vi "m1m3_putSample_HardpointMonitorData.vi"(8 "error in (no error)":errorcluster, 11 "HardpointMonitorData_Ctl":T1={"Timestamp"=0.0, "BreakawayLVDT[6]"=[0.0, 0.0, 0.0, 0.0, 0.0, 0.0], "DisplacementLVDT[6]"=[0.0, 0.0, 0.0, 0.0, 0.0, 0.0], "BreakawayPressure[6]"=[0.0, 0.0, 0.0, 0.0, 0.0, 0.0], "PressureSensor1[6]"=[0.0, 0.0, 0.0, 0.0, 0.0, 0.0], "PressureSensor2[6]"=[0.0, 0.0, 0.0, 0.0, 0.0, 0.0], "PressureSensor3[6]"=[0.0, 0.0, 0.0, 0.0, 0.0, 0.0]}) -> (0 "error out":errorcluster, 2 "function return":i32, 3 "HardpointMonitorData_Ctl out":T1)   [LabVIEW 2016, in "SALLV_m1m3.lvlib"]
doc: "int m1m3_shm_putSample_HardpointMonitorDataLV(m1m3_HardpointMonitorDataLV *HardpointMonitorData_Ctl );"
uses:
  SALLV_m1m3.lvlib
  DataTypes/HardpointMonitorData.ctl
  SALLV_m1m3.so
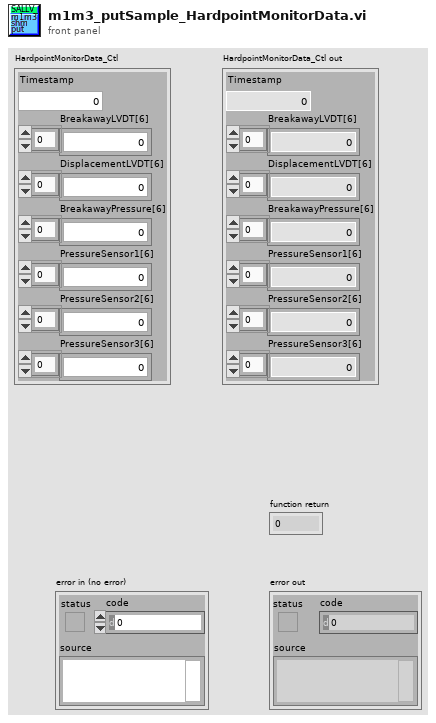
[diagram p1: front panel]
types:
  T1 = typedef "SALLV_m1m3.lvlib/HardpointMonitorData.ctl" = cluster{"Timestamp":dbl, "BreakawayLVDT[6]":sgl[], "DisplacementLVDT[6]":sgl[], "BreakawayPressure[6]":sgl[], "PressureSensor1[6]":sgl[], "PressureSensor2[6]":sgl[], "PressureSensor3[6]":sgl[]}
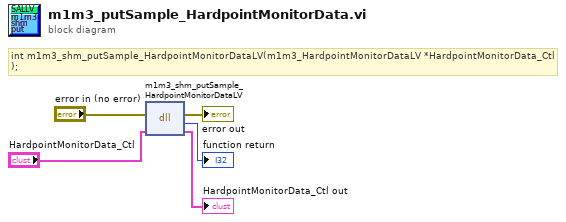
[diagram p0: block diagram]
diagram:
  # "int m1m3_shm_putSample_HardpointMonitorDataLV(m1m3_HardpointMonitorDataLV *HardpointMonitorData_Ctl );"
  n1 = dll-call lib="opt/CODE/SALLV_m1m3/SALLV_m1m3.*" fn="m1m3_shm_putSample_HardpointMonitorDataLV"(error in="error in (no error)", "HardpointMonitorData_Ctl"="HardpointMonitorData_Ctl") -> (error out=→"error out":errorcluster, →"function return":i32, "HardpointMonitorData_Ctl"=→"HardpointMonitorData_Ctl out":T1)  [unwired: 2 in, 1 out]
